vi "GSP_Manager_TCSLINK.vi"() -> ()   [LabVIEW 2015]
uses:
  SystemUtil/Command.ctl
  Log/LogItem.ctl
  TCSLINK_global.vi
panel:
  out "Command Recieved":bool
  in  "Lamp Cluster":T1
  out "M3":bool
  out "Guiding":bool
  out "ADC":u16(ring) caption="Dome Ind"
  out "Slewing":bool
  out "Comp Mirror":bool
  out "Tip/Tilt":bool
  out "Dome Moving":bool
  out "DEC":string
  out "RA":string
  out "Position Angle (E of N)":string
  out "Seeing":string
  out "Dome Shutter":string
  out "Mount El":string
  out "Humidity":string
  out "Wind Speed":string
  out "Wind Direction":string
  out "Focus":string
  out "Hour Angle":string
  out "Sidereal":string
  out "Dome Az":string
  out "Mount Az":string
  out "Pressure":string
  out "Outside Temp":string
  out "Airmass":string
  out "Rotator Angle":string
  out "UT Time":string
  out "Date":string
  out "Status":string="Shutdown"
  out "error out 2":errorcluster
  out "error out":errorcluster
  out "Rcv from TCS Q Out":refnum<queue>
  out "Send to TCS Q Out":refnum<queue>
  out "Rotator Location":string
  out "Last Error":errorcluster
  in  "CommandQ":string
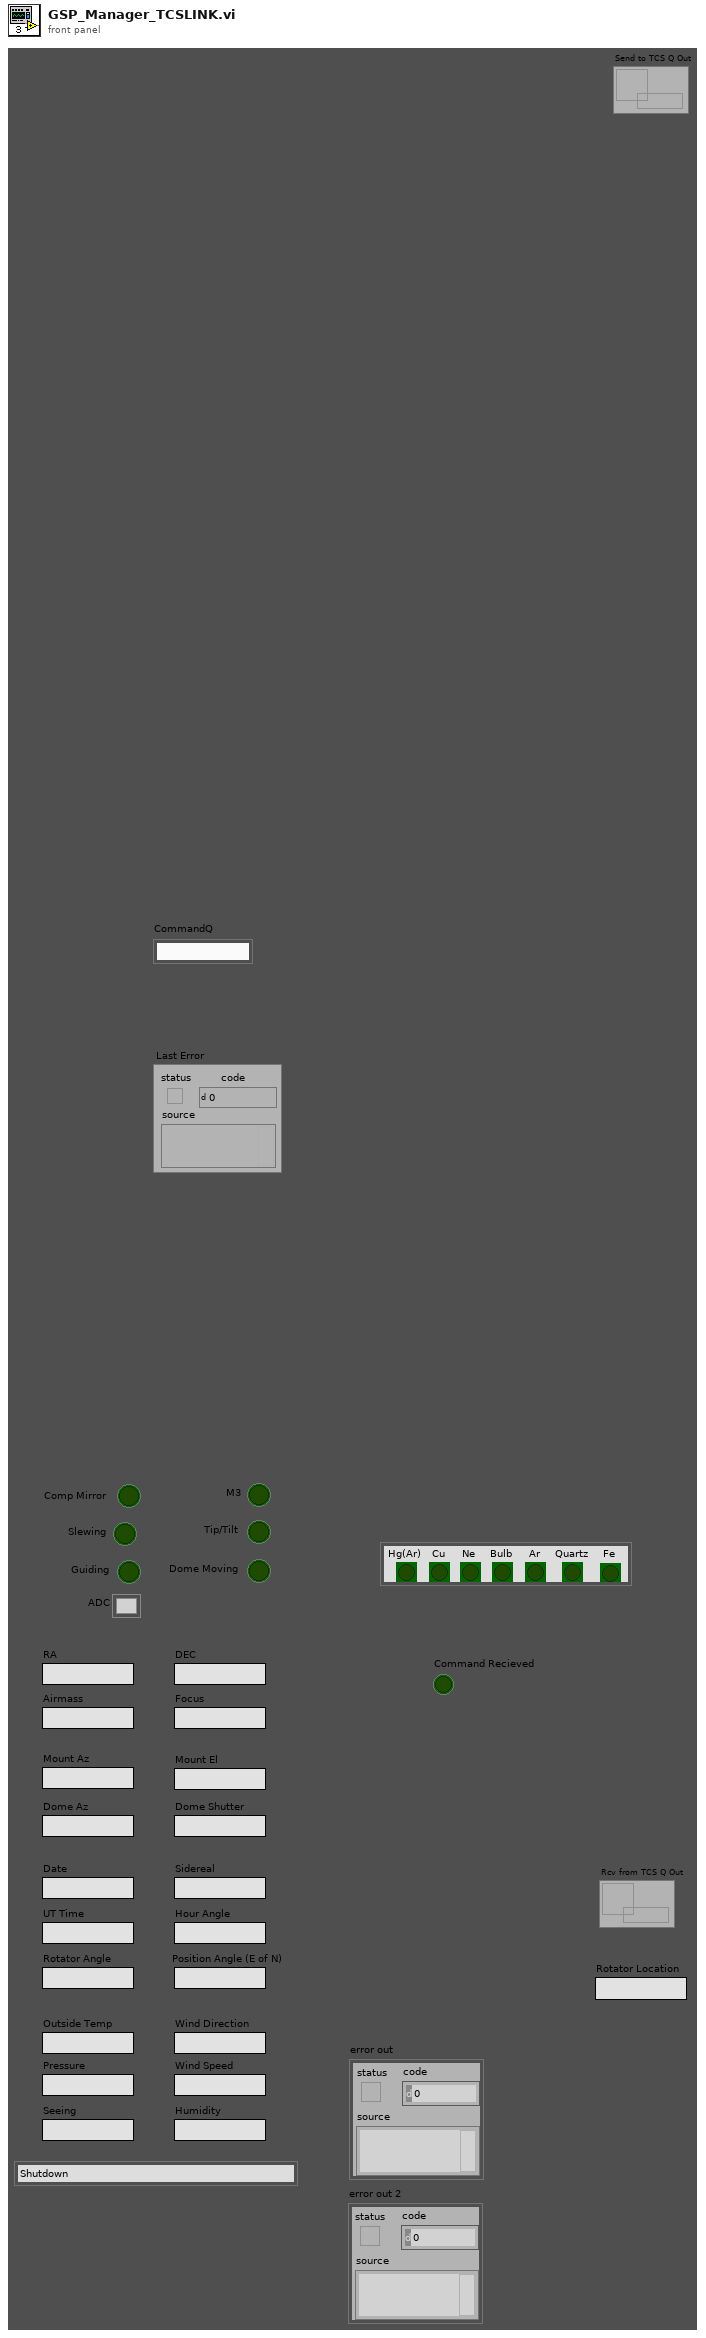
[diagram p1: front panel]
types:
  T1 = cluster{"Hg(Ar)":bool, "Cu":bool, "Ne":bool, "Ar":bool, "Quartz":bool, "Fe":bool, "Bulb":bool}
  T2 = typedef "Command.ctl" = cluster{"Command":string, "Parameter":string}
  T3 = typedef "LogItem.ctl" = cluster{"error in (no error)":errorcluster, "Source":string, "Comment ":string}
  T4 = enum16{"Launch", "Log", "Open", "Close", "Shutdown"}
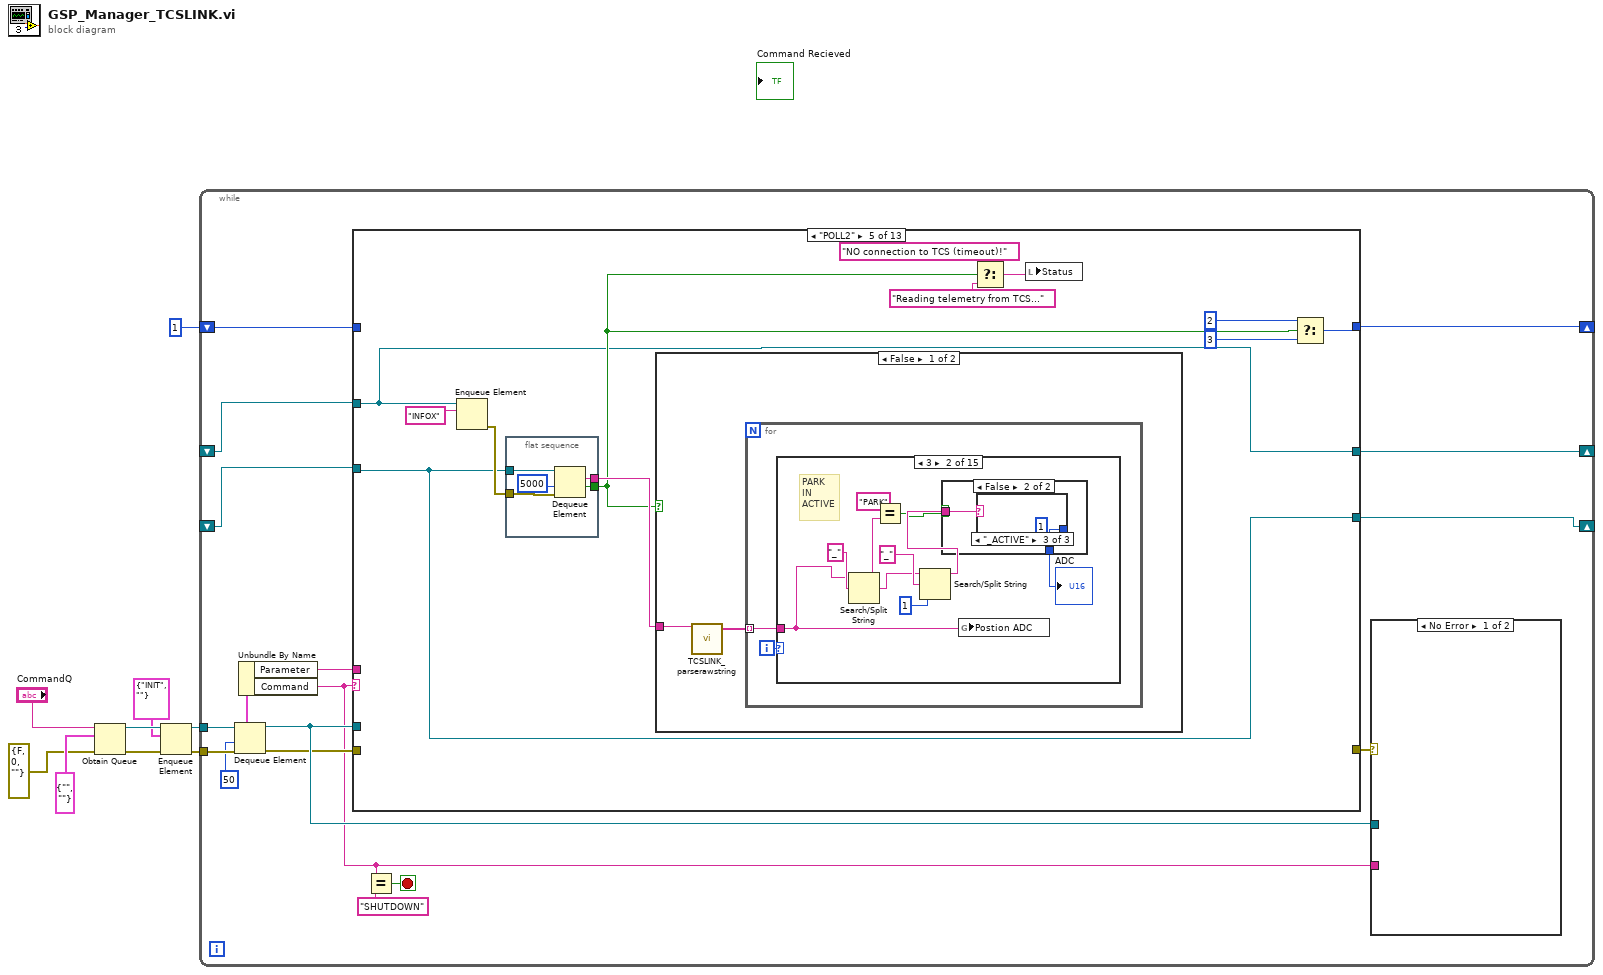
[diagram p0: block diagram]
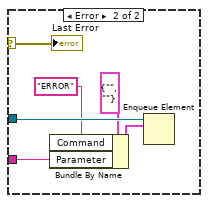
[diagram p2: hidden frame]
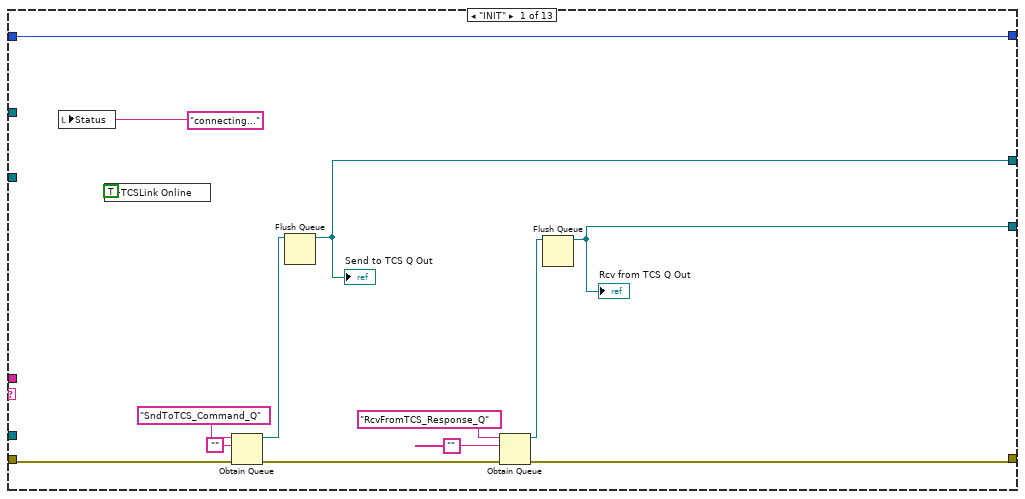
[diagram p3: hidden frame]
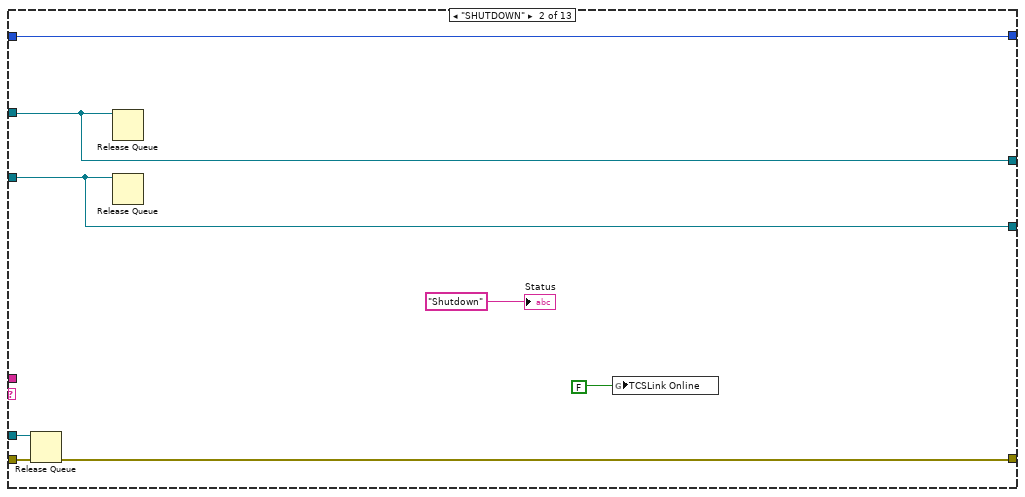
[diagram p4: hidden frame]
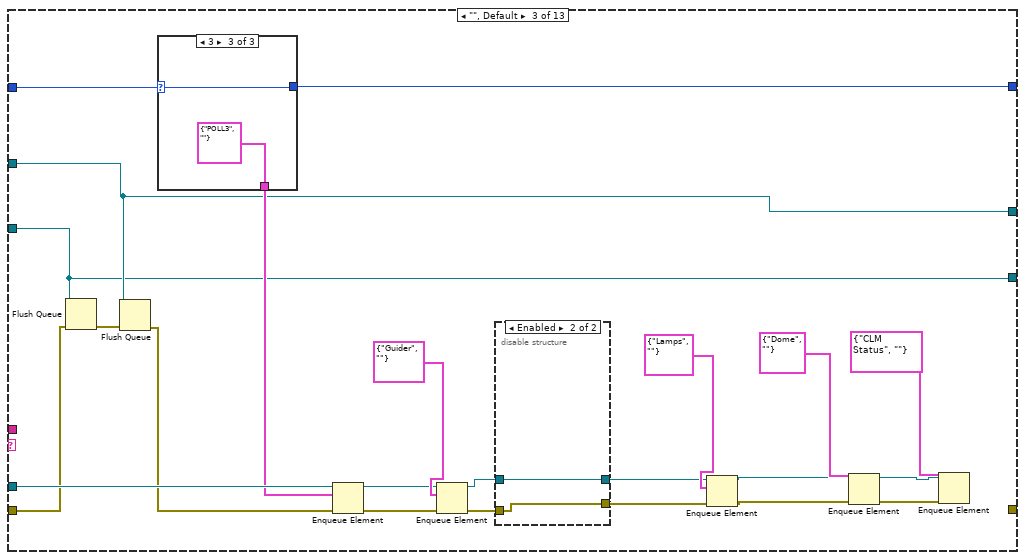
[diagram p5: hidden frame]
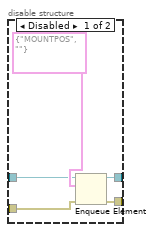
[diagram p6: hidden frame]
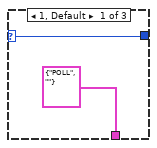
[diagram p7: hidden frame]
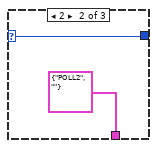
[diagram p8: hidden frame]
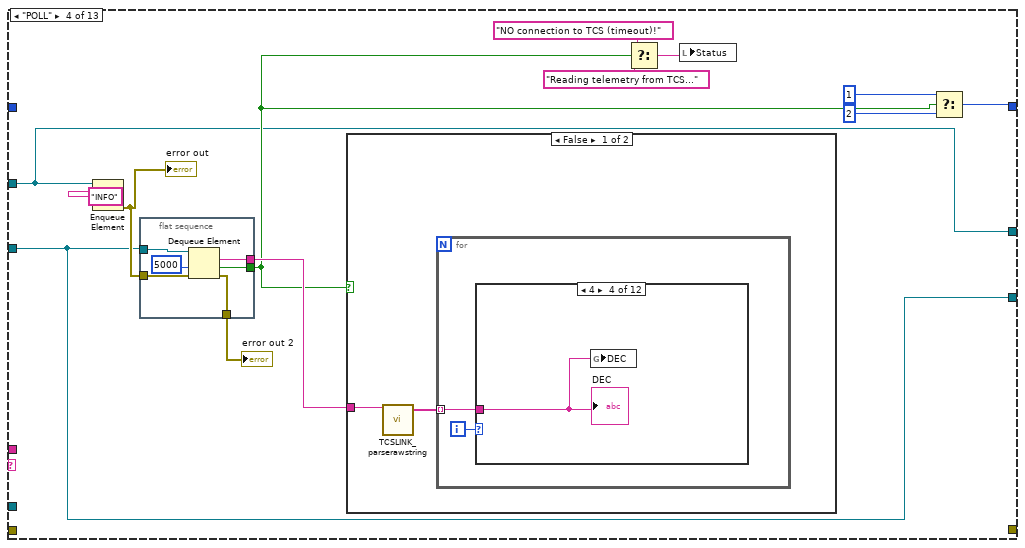
[diagram p9: hidden frame]
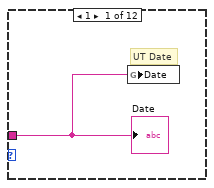
[diagram p10: hidden frame]
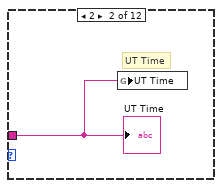
[diagram p11: hidden frame]
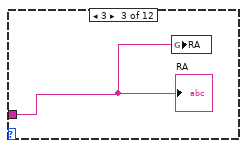
[diagram p12: hidden frame]
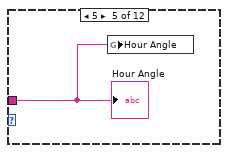
[diagram p13: hidden frame]
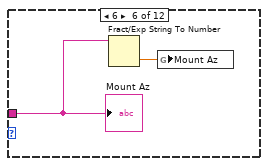
[diagram p14: hidden frame]
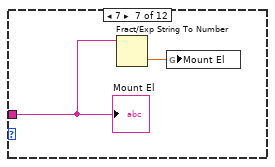
[diagram p15: hidden frame]
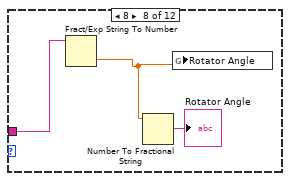
[diagram p16: hidden frame]
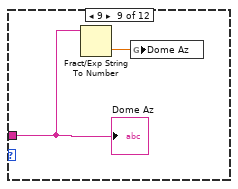
[diagram p17: hidden frame]
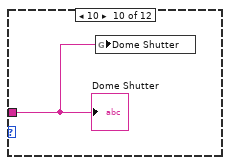
[diagram p18: hidden frame]
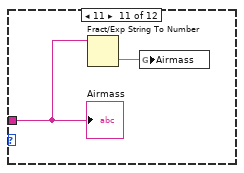
[diagram p19: hidden frame]
diagram:
  n1 = Obtain Queue(name (unnamed)="CommandQ", element data type=T2 {"Command"="", "Parameter"=""} ("Command"), error in (no error)=errorcluster {"status"=FALSE, "code"=0, "source"=""}) -> (queue out=w6:refnum<queue>, error out=w7:errorcluster)  [unwired: 2 in, 1 out]
  n2 = Enqueue Element(queue=w6, element=T2 {"Command"="INIT", "Parameter"=""}, error in (no error)=w7) -> (queue out=w9:refnum<queue>, error out=w8:errorcluster)  [unwired: 1 in, 1 out]
  n3 = while {
    tunnel: w9 -> [w26]
    tunnel: w8 -> [w25]
    shift-right: [w14] -> _
    shift-left: 1 ("timeout in ms (-1)") -> [w15]
    shift-right: [w12] -> _
    shift-left: _ -> [w10]
    shift-right: [w13] -> _
    shift-left: _ -> [w11]
    stop <- w18 stop-if-true
    n4 = Dequeue Element(queue=w26, timeout in ms (-1)=50, error in (no error)=w25) -> (queue out=w23:refnum<queue>, element=w20:T2, error out=w21:errorcluster)  [unwired: 1 out]
    n5 = Unbundle By Name(w20) -> ("Parameter"=w19:string, "Command"=w17:string)
    n6 = case shown="\"POLL2\"" w17 {
      selector: w17 -> [_ _ _ _ _ _ w216 _ _ _ _ _ _]
      tunnel: w21 -> [w40 w53 w75 _ _ _ _ _ _ _ _ _ _]
      tunnel: w23 -> [_ w52 w77 _ _ _ _ _ _ _ _ _ w394]
      tunnel: [w38 w50 _ _ _ _ _ _ _ _ _ _ _] -> w24
      tunnel: w19 -> [_ _ _ _ _ _ _ _ _ _ _ _ _]
      tunnel: w11 -> [_ w48 w70 w92 w132 w198 w221 w239 w258 w277 w293 w316 w391]
      tunnel: w10 -> [_ w47 w69 w91 w131 w197 w220 w238 w257 w276 w294 w317 w390]
      tunnel: w15 -> [w35 w49 w72 _ _ w196 w219 w237 w256 w275 _ w315 w392]
      tunnel: [w35 w49 w71 w95 w133 w196 w219 w237 w256 w275 w291 w315 w392] -> w14
      tunnel: [w34 w48 w70 w92 w132 w198 w221 w239 w258 w277 w293 w316 w391] -> w13
      tunnel: [w33 w47 w69 w91 w131 w197 w220 w238 w257 w276 w294 w317 w390] -> w12
      frame "INIT" {
        n7 = local write "Status"("connecting..." ("Value")) -> ()
        n8 = global write "TCSLINK_global.vi" "TCSLink Online"(TRUE) -> ()
        n9 = Obtain Queue(name (unnamed)="SndToTCS_Command_Q", element data type="", error in (no error)=w40) -> (queue out=w37:refnum<queue>, error out=w39:errorcluster)  [unwired: 2 in, 1 out]
        n10 = Flush Queue(queue=w37) -> (queue out=w34:refnum<queue>)  [unwired: 1 in, 2 out]
        "Send to TCS Q Out" <- w34
        n11 = Obtain Queue(name (unnamed)="RcvFromTCS_Response_Q", element data type="", error in (no error)=w39) -> (queue out=w36:refnum<queue>, error out=w38:errorcluster)  [unwired: 2 in, 1 out]
        n12 = Flush Queue(queue=w36) -> (queue out=w33:refnum<queue>)  [unwired: 1 in, 2 out]
        "Rcv from TCS Q Out" <- w33
      }
      frame "SHUTDOWN" {
        n13 = Release Queue(queue=w52, error in (no error)=w53) -> (error out=w50:errorcluster)  [unwired: 1 in, 2 out]
        n14 = Release Queue(queue=w48) -> ()  [unwired: 2 in, 3 out]
        n15 = Release Queue(queue=w47) -> ()  [unwired: 2 in, 3 out]
        n16 = global write "TCSLINK_global.vi" "TCSLink Online"(FALSE) -> ()
        "Status" <- "Shutdown" ("Value")
      }
      frame "", Default {
        n17 = Flush Queue(queue=w69, error in (no error)=w75) -> (error out=w74:errorcluster)  [unwired: 2 out]
        n18 = Flush Queue(queue=w70, error in (no error)=w74) -> (error out=w73:errorcluster)  [unwired: 2 out]
        n19 = case shown="3" w72 {
          selector: w72 -> [w85 w87 w89]
          tunnel: [T2 {"Command"="POLL", "Parameter"=""} ("element") T2 {"Command"="POLL2", "Parameter"=""} ("element") T2 {"Command"="POLL3", "Parameter"=""} ("element")] -> w76
          tunnel: [w85 w87 w89] -> w71
          frame 1, Default {
          }
          frame 2 {
          }
          frame 3 {
          }
        }
        n20 = Enqueue Element(queue=w77, element=w76, error in (no error)=w73) -> (queue out=w66:refnum<queue>, error out=w65:errorcluster)  [unwired: 1 in, 1 out]
        n21 = Enqueue Element(queue=w66, element=T2 {"Command"="Guider", "Parameter"=""}, error in (no error)=w65) -> (queue out=w58:refnum<queue>, error out=w57:errorcluster)  [unwired: 1 in, 1 out]
        n22 = disable-structure shown="Enabled" {
          disable-tunnel: w58 -> [w81 w84]
          disable-tunnel: w57 -> [w80 w83]
          disable-tunnel: [w79 w84] -> w56
          disable-tunnel: [w78 w83] -> w55
          frame Disabled {
            n23 = Enqueue Element(queue=w81, element=T2 {"Command"="MOUNTPOS", "Parameter"=""}, error in (no error)=w80) -> (queue out=w79:refnum<queue>, error out=w78:errorcluster)  [unwired: 1 in, 1 out]
          }
          frame Enabled {
          }
        }
        n24 = Enqueue Element(queue=w56, element=T2 {"Command"="Lamps", "Parameter"=""}, error in (no error)=w55) -> (queue out=w63:refnum<queue>, error out=w62:errorcluster)  [unwired: 1 in, 1 out]
        n25 = Enqueue Element(queue=w63, element=T2 {"Command"="Dome", "Parameter"=""}, error in (no error)=w62) -> (queue out=w60:refnum<queue>, error out=w59:errorcluster)  [unwired: 1 in, 1 out]
        n26 = Enqueue Element(queue=w60, element=T2 {"Command"="CLM Status", "Parameter"=""}, error in (no error)=w59) -> ()  [unwired: 1 in, 3 out]
      }
      frame "POLL" {
        n27 = Enqueue Element(queue=w92, element="INFO") -> (error out=w94:errorcluster)  [unwired: 2 in, 2 out]
        "error out" <- w94
        n28 = flat-sequence {
          tunnel: w91 -> [w108]
          tunnel: w94 -> [w107]
          tunnel: [w106] -> w99
          tunnel: [w105] -> w97
          tunnel: [w104] -> w93
          frame #0 {
            n29 = Dequeue Element(queue=w108, timeout in ms (-1)=5000, error in (no error)=w107) -> (element=w106:string, timed out?=w105:bool, error out=w104:errorcluster)  [unwired: 1 out]
          }
        }
        n30 = case shown="False" w97 {
          tunnel: w99 -> [w110 _]
          frame False {
            n31 = call "TCSLINK_parserawstring.vi"("Raw String"=w110) -> ("Array"=w111:string[])  [unwired: 4 in]
            n32 = for {
              tunnel: w111 -> [w112] mode=indexing
              i -> [w113]
              n33 = case shown="4" w113 {
                tunnel: w112 -> [w114 w115 w116 w117 w118 w120 w121 w125 w126 w128 w129 _]
                frame 1 {
                  # "UT Date"
                  n34 = global write "TCSLINK_global.vi" "Date"(w114) -> ()
                  "Date" <- w114
                }
                frame 2 {
                  # "UT Time"
                  n35 = global write "TCSLINK_global.vi" "UT Time"(w115) -> ()
                  "UT Time" <- w115
                }
                frame 3 {
                  n36 = global write "TCSLINK_global.vi" "RA"(w116) -> ()
                  "RA" <- w116
                }
                frame 4 {
                  n37 = global write "TCSLINK_global.vi" "DEC"(w117) -> ()
                  "DEC" <- w117
                }
                frame 5 {
                  n38 = global write "TCSLINK_global.vi" "Hour Angle"(w118) -> ()
                  "Hour Angle" <- w118
                }
                frame 6 {
                  n39 = Fract/Exp String To Number(string=w120) -> (number=w119:dbl)  [unwired: 3 in, 1 out]
                  n40 = global write "TCSLINK_global.vi" "Mount Az"(w119) -> ()
                  "Mount Az" <- w120
                }
                frame 7 {
                  n41 = Fract/Exp String To Number(string=w121) -> (number=w122:dbl)  [unwired: 3 in, 1 out]
                  n42 = global write "TCSLINK_global.vi" "Mount El"(w122) -> ()
                  "Mount El" <- w121
                }
                frame 8 {
                  n43 = Fract/Exp String To Number(string=w125) -> (number=w123:dbl)  [unwired: 3 in, 1 out]
                  n44 = Number To Fractional String(number=w123) -> (F-format string=→"Rotator Angle":string)  [unwired: 3 in]
                  n45 = global write "TCSLINK_global.vi" "Rotator Angle"(w123) -> ()
                }
                frame 9 {
                  n46 = Fract/Exp String To Number(string=w126) -> (number=w127:dbl)  [unwired: 3 in, 1 out]
                  n47 = global write "TCSLINK_global.vi" "Dome Az"(w127) -> ()
                  "Dome Az" <- w126
                }
                frame 10 {
                  n48 = global write "TCSLINK_global.vi" "Dome Shutter"(w128) -> ()
                  "Dome Shutter" <- w128
                }
                frame 11 {
                  n49 = Fract/Exp String To Number(string=w129) -> (number=w130:dbl)  [unwired: 3 in, 1 out]
                  n50 = global write "TCSLINK_global.vi" "Airmass"(w130) -> ()
                  "Airmass" <- w129
                }
                frame Default {
                }
              }
            }
          }
          frame True {
          }
        }
        n51 = Select(t="NO connection to TCS (timeout)!" ("Value"), s=w97, f="Reading telemetry from TCS...") -> (s? t:f=w101:string)
        n52 = local write "Status"(w101) -> ()
        n53 = Select(t=i8 1, s=w97, f=i8 2) -> (s? t:f=w95:i8)
        "error out 2" <- w93
      }
      frame "POLL2" {
        n54 = Enqueue Element(queue=w132, element="INFOX") -> (error out=w138:errorcluster)  [unwired: 2 in, 2 out]
        n55 = flat-sequence {
          tunnel: w131 -> [w146]
          tunnel: w138 -> [w145]
          tunnel: [w144] -> w137
          tunnel: [w143] -> w134
          frame #0 {
            n56 = Dequeue Element(queue=w146, timeout in ms (-1)=5000, error in (no error)=w145) -> (element=w144:string, timed out?=w143:bool)  [unwired: 2 out]
          }
        }
        n57 = case shown="False" w134 {
          tunnel: w137 -> [w148 _]
          frame False {
            n58 = call "TCSLINK_parserawstring.vi"("Raw String"=w148) -> ("Array"=w149:string[])  [unwired: 4 in]
            n59 = for {
              tunnel: w149 -> [w150] mode=indexing
              i -> [w151]
              n60 = case shown="3" w151 {
                tunnel: w150 -> [w152 w161 w169 w171 w173 w175 w177 w179 w181 w182 w188 _ w193 w195 _]
                frame 2 {
                  n61 = global write "TCSLINK_global.vi" "Sidereal Time"(w152) -> ()
                  "Sidereal" <- w152
                }
                frame 3 {
                  # "PARK \nIN\nACTIVE"
                  n62 = Search/Split String(string=w161, search string/char (-)="_" ("Comment")) -> (substring before match=w154:string, match + rest of string=w157:string)  [unwired: 1 in, 1 out]
                  n63 = Equal?(x="PARK", y=w154) -> (x = y?=w153:bool)
                  n64 = Search/Split String(string=w157, search string/char (-)="_" ("Comment"), offset (0)=1) -> (substring before match=w158:string)  [unwired: 2 out]
                  n65 = case shown="False" w153 {
                    tunnel: [0 w165] -> w160
                    tunnel: w158 -> [_ w164]
                    frame True {
                    }
                    frame False {
                      n66 = case shown="\"_ACTIVE\"" w164 {
                        tunnel: [0 2 1] -> w165
                        frame "PARK", Default {
                        }
                        frame "_DONE" {
                        }
                        frame "_ACTIVE" {
                        }
                      }
                    }
                  }
                  "ADC" <- w160
                  n67 = global write "TCSLINK_global.vi" "Postion ADC"(w161) -> ()
                }
                frame 4 {
                  n68 = Fract/Exp String To Number(string=w169) -> (number=w170:dbl)  [unwired: 3 in, 1 out]
                  n69 = global write "TCSLINK_global.vi" "Focus"(w170) -> ()
                  "Focus" <- w169
                }
                frame 5 {
                  n70 = Fract/Exp String To Number(string=w171) -> (number=w172:dbl)  [unwired: 3 in, 1 out]
                  n71 = global write "TCSLINK_global.vi" "Outside Temp"(w172) -> ()
                  "Outside Temp" <- w171
                }
                frame 6 {
                  n72 = Fract/Exp String To Number(string=w173) -> (number=w174:dbl)  [unwired: 3 in, 1 out]
                  n73 = global write "TCSLINK_global.vi" "Humidity"(w174) -> ()
                  "Humidity" <- w173
                }
                frame 7 {
                  n74 = Fract/Exp String To Number(string=w175) -> (number=w176:dbl)  [unwired: 3 in, 1 out]
                  n75 = global write "TCSLINK_global.vi" "Pressure"(w176) -> ()
                  "Pressure" <- w175
                }
                frame 8 {
                  n76 = Fract/Exp String To Number(string=w177) -> (number=w178:dbl)  [unwired: 3 in, 1 out]
                  n77 = global write "TCSLINK_global.vi" "Wind Direction"(w178) -> ()
                  "Wind Direction" <- w177
                }
                frame 9 {
                  n78 = Fract/Exp String To Number(string=w179) -> (number=w180:dbl)  [unwired: 3 in, 1 out]
                  n79 = global write "TCSLINK_global.vi" "Wind Speed"(w180) -> ()
                  "Wind Speed" <- w179
                }
                frame 10 {
                  n80 = global write "TCSLINK_global.vi" "ObsRA"(w181) -> ()
                }
                frame 11 {
                  n81 = global write "TCSLINK_global.vi" "ObsDEC"(w182) -> ()
                }
                frame 16 {
                  w186 = 360.0 ("x")
                  n82 = Fract/Exp String To Number(string=w188) -> (number=w183:dbl)  [unwired: 3 in, 1 out]
                  n83 = Greater?(x=w183, y=w186) -> (0:w187:bool)
                  n84 = case shown="False" w187 {
                    tunnel: w183 -> [w189 w192]
                    tunnel: w186 -> [_ w191]
                    tunnel: [w189 w190] -> w184
                    frame False {
                    }
                    frame True {
                      n85 = Subtract(x=w192, y=w191) -> (x-y=w190:dbl)
                    }
                  }
                  n86 = global write "TCSLINK_global.vi" "Position Angle"(w184) -> ()
                  n87 = Format Into String(w184) -> (resulting string=→"Position Angle (E of N)":string)  [unwired: 3 in, 1 out]
                }
                frame 15 {
                }
                frame 18 {
                  n88 = Fract/Exp String To Number(string=w193) -> (number=w194:dbl)  [unwired: 3 in, 1 out]
                  n89 = global write "TCSLINK_global.vi" "Seeing"(w194) -> ()
                  "Seeing" <- w193
                }
                frame 999 {
                  n90 = global write "TCSLINK_global.vi" "Rotator Location"(w195) -> ()
                  "Rotator Location" <- w195
                }
                frame Default {
                }
              }
            }
          }
          frame True {
          }
        }
        n91 = Select(t="NO connection to TCS (timeout)!" ("Value"), s=w134, f="Reading telemetry from TCS...") -> (s? t:f=w140:string)
        n92 = local write "Status"(w140) -> ()
        n93 = Select(t=i8 2, s=w134, f=i8 3) -> (s? t:f=w133:i8)
      }
      frame "Guider" {
        n94 = Enqueue Element(queue=w198, element="GUIDER STATUS") -> (error out=w201:errorcluster)  [unwired: 2 in, 2 out]
        n95 = flat-sequence {
          tunnel: w197 -> [w206]
          tunnel: w201 -> [w205]
          tunnel: [w204] -> w200
          tunnel: [w203] -> w199
          frame #0 {
            n96 = Dequeue Element(queue=w206, timeout in ms (-1)=5000, error in (no error)=w205) -> (element=w204:string, timed out?=w203:bool)  [unwired: 2 out]
          }
        }
        n97 = case shown="False" w199 {
          tunnel: w200 -> [w208 _]
          frame False {
            n98 = call "TCSLINK_parserawstring.vi"("Raw String"=w208) -> ("Array"=w209:string[])  [unwired: 4 in]
            n99 = for {
              tunnel: w209 -> [w211] mode=indexing
              i -> [w210]
              n100 = case shown="1" w210 {
                tunnel: w211 -> [_ w213]
                frame Default {
                }
                frame 1 {
                  n101 = Equal?(x="ENABLE", y=w213) -> (x = y?=→"Guiding":bool)
                }
              }
            }
          }
          frame True {
          }
        }
      }
      frame "CLM" {
        n102 = call <vilib>:"Space Constant.vi"() -> ("String"=w217:string)
        n103 = Concatenate Strings("CLM" ("element"), w217, w216) -> (w215:string)
        n104 = Enqueue Element(queue=w221, element=w215) -> (error out=w224:errorcluster)  [unwired: 2 in, 2 out]
        n105 = flat-sequence {
          tunnel: w220 -> [w228]
          tunnel: w224 -> [w227]
          tunnel: [w226] -> w223
          tunnel: [w225] -> w222
          frame #0 {
            n106 = Dequeue Element(queue=w228, timeout in ms (-1)=5000, error in (no error)=w227) -> (element=w226:string, timed out?=w225:bool)  [unwired: 2 out]
          }
        }
        n107 = case shown="False" w222 {
          tunnel: w223 -> [w230 _]
          frame False {
            n108 = call "TCSLINK_parserawstring.vi"("Raw String"=w230) -> ("Array"=w231:string[])  [unwired: 4 in]
            n109 = for {
              tunnel: w231 -> [w233] mode=indexing
              i -> [w232]
              n110 = case shown="0" w232 {
                tunnel: w233 -> [_ w236]
                frame Default {
                }
                frame 0 {
                  n111 = Equal?(x="ACTIVE", y=w236) -> (x = y?=w234:bool)
                  n112 = local write "Command Recieved"(w234) -> ()
                }
              }
            }
          }
          frame True {
          }
        }
      }
      frame "CLM Status" {
        n113 = Enqueue Element(queue=w239, element="CLM STATUS") -> (error out=w242:errorcluster)  [unwired: 2 in, 2 out]
        n114 = flat-sequence {
          tunnel: w238 -> [w247]
          tunnel: w242 -> [w246]
          tunnel: [w245] -> w241
          tunnel: [w244] -> w240
          frame #0 {
            n115 = Dequeue Element(queue=w247, timeout in ms (-1)=5000, error in (no error)=w246) -> (element=w245:string, timed out?=w244:bool)  [unwired: 2 out]
          }
        }
        n116 = case shown="False" w240 {
          tunnel: w241 -> [w249 _]
          frame False {
            n117 = call "TCSLINK_parserawstring.vi"("Raw String"=w249) -> ("Array"=w250:string[])  [unwired: 4 in]
            n118 = for {
              tunnel: w250 -> [w252] mode=indexing
              i -> [w251]
              n119 = case shown="1" w251 {
                tunnel: w252 -> [_ w254]
                frame Default {
                }
                frame 1 {
                  n120 = Equal?(x="IN", y=w254) -> (x = y?=w253:bool)
                  "Comp Mirror" <- w253
                  n121 = global write "TCSLINK_global.vi" "Comp Mirror"(w253) -> ()
                }
              }
            }
          }
          frame True {
          }
        }
      }
      frame "Dome" {
        n122 = Enqueue Element(queue=w258, element="WHITESPOT STATUS") -> (error out=w261:errorcluster)  [unwired: 2 in, 2 out]
        n123 = flat-sequence {
          tunnel: w257 -> [w266]
          tunnel: w261 -> [w265]
          tunnel: [w264] -> w260
          tunnel: [w263] -> w259
          frame #0 {
            n124 = Dequeue Element(queue=w266, timeout in ms (-1)=5000, error in (no error)=w265) -> (element=w264:string, timed out?=w263:bool)  [unwired: 2 out]
          }
        }
        n125 = case shown="False" w259 {
          tunnel: w260 -> [w268 _]
          frame False {
            n126 = call "TCSLINK_parserawstring.vi"("Raw String"=w268) -> ("Array"=w269:string[])  [unwired: 4 in]
            n127 = for {
              tunnel: w269 -> [w271] mode=indexing
              i -> [w270]
              n128 = case shown="1" w270 {
                tunnel: w271 -> [_ w274]
                frame Default {
                }
                frame 1 {
                  n129 = Decimal String To Number(string=w274) -> (number=w272:i32)  [unwired: 2 in, 1 out]
                  n130 = Greater Than 0?(x=w272) -> (x > 0?=w273:bool)
                  n131 = global write "TCSLINK_global.vi" "Dome Percent"(w272) -> ()
                  n132 = global write "TCSLINK_global.vi" "Dome"(w273) -> ()
                }
              }
            }
          }
          frame True {
          }
        }
      }
      frame "MOUNTPOS" {
        n133 = Enqueue Element(queue=w277, element="") -> (error out=w280:errorcluster)  [unwired: 2 in, 2 out]
        n134 = flat-sequence {
          tunnel: w276 -> [w285]
          tunnel: w280 -> [w284]
          tunnel: [w283] -> w279
          tunnel: [w282] -> w278
          frame #0 {
            n135 = Dequeue Element(queue=w285, timeout in ms (-1)=5000, error in (no error)=w284) -> (element=w283:string, timed out?=w282:bool)  [unwired: 2 out]
          }
        }
        n136 = case shown="False" w278 {
          tunnel: w279 -> [w287 _]
          frame False {
            n137 = call "TCSLINK_parserawstring.vi"("Raw String"=w287) -> ("Array"=w288:string[])  [unwired: 4 in]
            n138 = for {
              tunnel: w288 -> [w290] mode=indexing
              i -> [w289]
              n139 = case shown="1" w289 {
                tunnel: w290 -> [_ _]
                frame Default {
                }
                frame 1 {
                }
              }
            }
          }
          frame True {
          }
        }
      }
      frame "POLL3" {
        n140 = Enqueue Element(queue=w293, element="ROTSPOS") -> (error out=w299:errorcluster)  [unwired: 2 in, 2 out]
        n141 = flat-sequence {
          tunnel: w294 -> [w306]
          tunnel: w299 -> [w305]
          tunnel: [w304] -> w298
          tunnel: [w303] -> w295
          frame #0 {
            n142 = Dequeue Element(queue=w306, timeout in ms (-1)=5000, error in (no error)=w305) -> (element=w304:string, timed out?=w303:bool)  [unwired: 2 out]
          }
        }
        n143 = case shown="False" w295 {
          tunnel: w298 -> [w309 _]
          frame False {
            n144 = call "TCSLINK_parserawstring.vi"("Raw String"=w309) -> ("Array"=w308:string[])  [unwired: 4 in]
            n145 = for {
              tunnel: w308 -> [w310] mode=indexing
              i -> [w311]
              n146 = case shown="6" w311 {
                tunnel: w310 -> [w313 _ _ _ _ _]
                frame 6 {
                  n147 = Equal?(x="5", y=w313) -> (x = y?=→"M3":bool)
                }
                frame 8 {
                }
                frame Default {
                }
                frame 3 {
                }
                frame 4 {
                }
                frame 5 {
                }
              }
            }
          }
          frame True {
          }
        }
        n148 = Select(t="NO connection to TCS (timeout)!" ("Value"), s=w295, f="Reading telemetry from TCS...") -> (s? t:f=w292:string)
        n149 = local write "Status"(w292) -> ()
        n150 = Select(t=i8 3, s=w295, f=i8 1) -> (s? t:f=w291:i8)
      }
      frame "Lamps" {
        n151 = property on="Lamp Cluster" class="Clust (strict)"() -> ("Controls[]"=w318:refnum<vi>[])  [unwired: 2 in, 2 out]
        n152 = for {
          tunnel: w317 -> [w325]
          tunnel: w316 -> [w326]
          tunnel: w318 -> [w324] mode=indexing
          w328 = " " ("string")
          n153 = property class="Ctl"(reference=w324) -> ("Label.Text"=w321:string)  [unwired: 1 in, 2 out]
          n154 = case shown="\"Fe\"" w321 {
            tunnel: ["L1" ("string") "L4" ("string") "L2" ("string") "L5" "L3" ("string") "L9" ("string") "L11" ("string") ""] -> w320
            frame "Hg(Ar)" {
            }
            frame "Cu" {
            }
            frame "Ne" {
            }
            frame "Fe" {
            }
            frame "Ar" {
            }
            frame "Quartz" {
            }
            frame "Bulb" {
            }
            frame "", Default {
            }
          }
          n155 = Concatenate Strings("LAMP", w328, w320, w328, "STATUS", w328) -> (w327:string)
          n156 = Enqueue Element(queue=w326, element=w327) -> ()  [unwired: 2 in, 3 out]
          n157 = Dequeue Element(queue=w325, timeout in ms (-1)=2000) -> (element=w323:string)  [unwired: 1 in, 3 out]
          n158 = call "TCSLINK_parserawstring.vi"("Raw String"=w323) -> ("Array"=w322:string[])  [unwired: 4 in]
          n159 = case shown="\"Quartz\"" w321 {
            tunnel: w322 -> [w331 w337 w343 w349 w355 w361 w376 _]
            frame "Hg(Ar)" {
              n160 = for {
                tunnel: w331 -> [w332] mode=indexing
                i -> [w333]
                n161 = case shown="2" w333 {
                  tunnel: w332 -> [_ w336]
                  frame 0, Default {
                  }
                  frame 2 {
                    n162 = Equal?(x=w336, y="ON") -> (x = y?=w334:bool)
                    n163 = global write "TCSLINK_global.vi" "Hg(Ar)"(w334) -> ()
                  }
                }
              }
            }
            frame "Cu" {
              n164 = for {
                tunnel: w337 -> [w338] mode=indexing
                i -> [w339]
                n165 = case shown="0, Default" w339 {
                  tunnel: w338 -> [_ w342]
                  frame 0, Default {
                  }
                  frame 2 {
                    n166 = Equal?(x=w342, y="ON") -> (x = y?=w340:bool)
                    n167 = global write "TCSLINK_global.vi" "Cu"(w340) -> ()
                  }
                }
              }
            }
            frame "Ne" {
              n168 = for {
                tunnel: w343 -> [w344] mode=indexing
                i -> [w345]
                n169 = case shown="2" w345 {
                  tunnel: w344 -> [_ w348]
                  frame 0, Default {
                  }
                  frame 2 {
                    n170 = Equal?(x=w348, y="ON") -> (x = y?=w346:bool)
                    n171 = global write "TCSLINK_global.vi" "Ne"(w346) -> ()
                  }
                }
              }
            }
            frame "Fe" {
              n172 = for {
                tunnel: w349 -> [w350] mode=indexing
                i -> [w351]
                n173 = case shown="0, Default" w351 {
                  tunnel: w350 -> [_ w354]
                  frame 0, Default {
                  }
                  frame 2 {
                    n174 = Equal?(x=w354, y="ON") -> (x = y?=w352:bool)
                    n175 = global write "TCSLINK_global.vi" "Fe"(w352) -> ()
                  }
                }
              }
            }
            frame "Ar" {
              n176 = for {
                tunnel: w355 -> [w356] mode=indexing
                i -> [w357]
                n177 = case shown="0, Default" w357 {
                  tunnel: w356 -> [_ w360]
                  frame 0, Default {
                  }
                  frame 2 {
                    n178 = Equal?(x=w360, y="ON") -> (x = y?=w358:bool)
                    n179 = global write "TCSLINK_global.vi" "Ar"(w358) -> ()
                  }
                }
              }
            }
            frame "Quartz" {
              n180 = for {
                tunnel: w361 -> [w362] mode=indexing
                i -> [w363]
                n181 = case shown="4" w363 {
                  tunnel: w362 -> [_ w369 w375]
                  frame 0, Default {
                  }
                  frame 2 {
                    n182 = global read "TCSLINK_global.vi" "Quartz Percent"() -> (w364:i8)
                    n183 = Equal?(x=w369, y="ON") -> (x = y?=w367:bool)
                    n184 = global write "TCSLINK_global.vi" "Quartz"(w367) -> ()
                    n185 = Select(t=w364, s=w367, f=0) -> (s? t:f=w365:i32)
                    n186 = global write "TCSLINK_global.vi" "Quartz Percent"(w365) -> ()
                  }
                  frame 4 {
                    n187 = Decimal String To Number(string=w375) -> (number=w374:i32)  [unwired: 2 in, 1 out]
                    n188 = global read "TCSLINK_global.vi" "Quartz"() -> (w373:bool)
                    n189 = Round To Nearest(number=w374) -> (nearest integer value=w372:i32)
                    n190 = Select(t=w372, s=w373, f=0) -> (s? t:f=w371:i32)
                    n191 = global write "TCSLINK_global.vi" "Quartz Percent"(w371) -> ()
                  }
                }
              }
            }
            frame "Bulb" {
              n192 = for {
                tunnel: w376 -> [w377] mode=indexing
                i -> [w378]
                n193 = case shown="0, Default" w378 {
                  tunnel: w377 -> [_ w381]
                  frame 0, Default {
                  }
                  frame 2 {
                    n194 = Equal?(x=w381, y="ON") -> (x = y?=w379:bool)
                    n195 = global write "TCSLINK_global.vi" "Bulb"(w379) -> ()
                  }
                }
              }
            }
            frame "", Default {
            }
          }
        }
      }
      frame "ERROR" {
        n196 = local read "Last Error"() -> (w395:errorcluster)
        n197 = Unbundle By Name(w395) -> ("code"=w401:i32)
        n198 = Bundle By Name(cluster=T3 {"error in (no error)"={"status"=FALSE, "code"=0, "source"=""}, "Source"="", "Comment "=""} ("Log"), "error in (no error)"=w395, "Source"="TCSLink Manager") -> (w398:T3)
        n199 = call "GSP_Logger_Handler.vi"("Log"=w398, "Actions"=T4."Log") -> ()  [unwired: 5 in, 1 out]
        n200 = case shown="0, Default" w401 {
          tunnel: w395 -> [_]
          tunnel: [w408] -> w396
          tunnel: w394 -> [w407]
          tunnel: [w409] -> w393
          tunnel: w391 -> [w405]
          tunnel: w390 -> [w404]
          frame 0, Default {
            n201 = Release Queue(queue=w405) -> ()  [unwired: 2 in, 3 out]
            n202 = Release Queue(queue=w404) -> ()  [unwired: 2 in, 3 out]
            n203 = local write "Status"("Error" ("Value")) -> ()
            n204 = Enqueue Element(queue=w407, element=T2 {"Command"="INIT", "Parameter"=""}) -> (queue out=w409:refnum<queue>, error out=w408:errorcluster)  [unwired: 2 in, 1 out]
          }
        }
        n205 = case shown="Error" w396 {
          tunnel: w393 -> [_ w403]
          frame No Error {
          }
          frame Error {
            n206 = Enqueue Element At Opposite End(queue=w403, element=T2 {"Command"="SHUTDOWN", "Parameter"=""}) -> ()  [unwired: 2 in, 3 out]
          }
        }
      }
    }
    n207 = Equal?(x=w17, y="SHUTDOWN") -> (x = y?=w18:bool)
    n208 = case shown="No Error" w24 {
      selector: w24 -> [_ w31]
      tunnel: w23 -> [_ w32]
      tunnel: w17 -> [_ w28]
      frame No Error {
      }
      frame Error {
        n209 = Bundle By Name(cluster=T2 {"Command"="", "Parameter"=""} ("element"), "Command"="ERROR" ("element"), "Parameter"=w28) -> (w30:T2)
        n210 = Enqueue Element(queue=w32, element=w30) -> ()  [unwired: 2 in, 3 out]
        "Last Error" <- w31
      }
    }
  }
